vi "ConfigTrigger.vi"(8 "error in (no error)":errorcluster, 11 "ClassIn":refnum<class "NiPxi6733.lvclass">) -> (0 "error out":errorcluster, 3 "ClassOut":refnum<class "NiPxi6733.lvclass">)   [LabVIEW 2014, in "FGenPlugins.lvlib" / "NiPxi6733.lvclass"]
uses:
  NiPxi6733.lvclass
  <vilib>/DAQmx/configure/trigger.llb/DAQmx Start Trigger (None).vi
  <vilib>/DAQmx/configure/trigger.llb/DAQmx Start Trigger (Digital Edge).vi
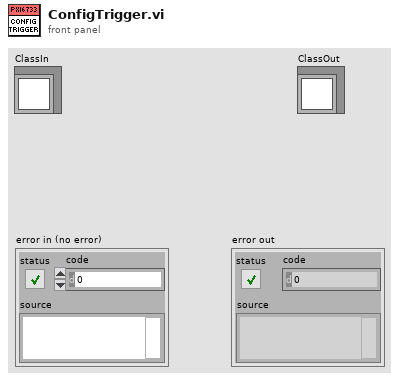
[diagram p1: front panel]
types:
  T1 = typedef "NISTFGenPlugins.lvlib/NISTFGenPluginsBase.lvclass/TriggerParams.ctl" = cluster{"eTrigger":u16, "eEdge":u16, "sSource":string}
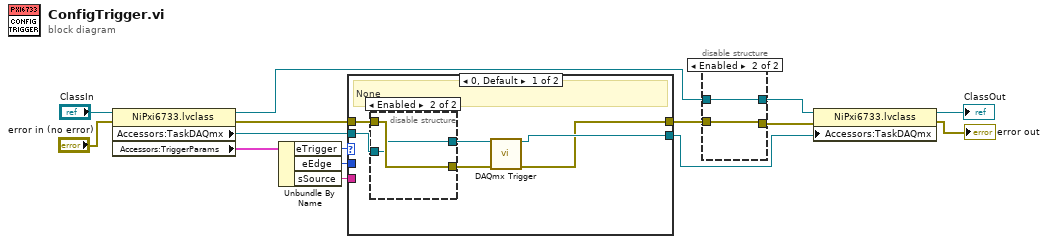
[diagram p0: block diagram]
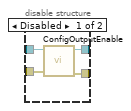
[diagram p2: hidden frame]
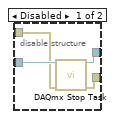
[diagram p3: hidden frame]
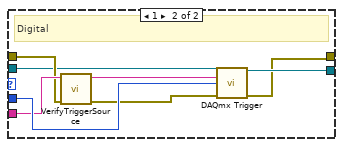
[diagram p4: hidden frame]
diagram:
  n1 = property class="NiPxi6733.lvclass"(reference="ClassIn", error in="error in (no error)") -> (reference out=w1:refnum<class "NiPxi6733.lvclass">, error out=w12:errorcluster, "Accessors:TaskDAQmx"=w14:refnum<k21>, "Accessors:TriggerParams"=w8:T1)
  n2 = Unbundle By Name(w8) -> ("eTrigger"=w7:u16, "eEdge"=w6:u16, "sSource"=w5:string)
  n3 = case shown="0, Default" w7 {
    tunnel: w14 -> [w19 w29]
    tunnel: w12 -> [w17 w32]
    tunnel: [w21 w35] -> w11
    tunnel: [w20 w31] -> w4
    tunnel: w6 -> [_ w34]
    tunnel: w5 -> [_ w33]
    frame 0, Default {
      # "None"
      n4 = disable-structure shown="Enabled" {
        disable-tunnel: w19 -> [w25 w26]
        disable-tunnel: [w24 w26] -> w18
        disable-tunnel: w17 -> [w23 w27]
        disable-tunnel: [w22 w27] -> w16
        frame Disabled {
          n5 = call <vilib>:"DAQmx Stop Task.vi"("task/channels in"=w25, "error in"=w23) -> ("task out"=w24:refnum<k21>, "error out"=w22:errorcluster)  [unwired: 12 in]
        }
        frame Enabled {
        }
      }
      n6 = call-poly <vilib>:"DAQmx Trigger.vi"("task/channels in"=w18, "error in"=w16) -> ("task out"=w21:refnum<k21>, "error out"=w20:errorcluster)  [unwired: 12 in]
    }
    frame 1 {
      # "Digital"
      n7 = call "VerifyTriggerSource.vi"("error in (no error)"=w32, "TriggerSource"=w33) -> ("error out"=w28:errorcluster, "DAQmx Terminal"=w30:tag)  [unwired: 8 in]
      n8 = call-poly <vilib>:"DAQmx Trigger.vi"("task/channels in"=w29, "source"=w30, "edge"=w34, "error in"=w28) -> ("task out"=w35:refnum<k21>, "error out"=w31:errorcluster)  [unwired: 10 in]
    }
  }
  n9 = disable-structure shown="Enabled" {
    disable-tunnel: w4 -> [w39 w40]
    disable-tunnel: [w38 w40] -> w3
    disable-tunnel: [w37 w41] -> w2
    disable-tunnel: w1 -> [w36 w41]
    frame Disabled {
      n10 = call-dynamic "ConfigOutputEnable.vi"("error in (no error)"=w39, "ClassIn"=w36) -> ("error out"=w38:errorcluster, "ClassOut"=w37:refnum<class "NiPxi6733.lvclass">)  [unwired: 8 in]
    }
    frame Enabled {
    }
  }
  n11 = property class="NiPxi6733.lvclass"(reference=w2, error in=w3, "Accessors:TaskDAQmx"=w11) -> (reference out=→"ClassOut":refnum<class "NiPxi6733.lvclass">, error out=→"error out":errorcluster)
